vi "主函数.vi"() -> ()   [LabVIEW 2020]
doc: "UDP协议与TCP的区别在于UDP不包括发送数据包信息的错误检查，因此无法保证接收端是否已接收所发数据。\n\nUDP可用于“广播”数据至整个网络，只需指定可包括全部的IP地址(255.255.255.255)以便发送信息至整个网络。 由于路由器或其他网络硬件通常拒绝转发超过一定点的数据，在实际应用中广播范围可能存在限制。"
panel:
  in  "停止输入":bool
  out "数据状态":string
  out "当前采集数据IP地址":string
  out "输出波形":waveform(i32)[](graph)
  in  "输出文件夹名称":path
  in  "数据采集卡IP地址":string
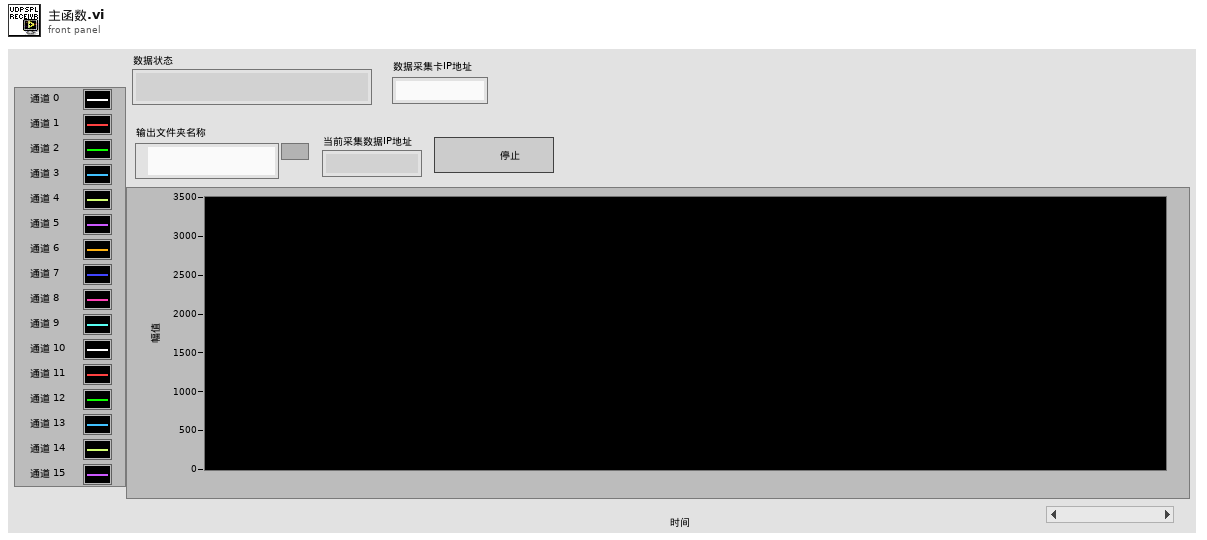
[diagram p1: front panel]
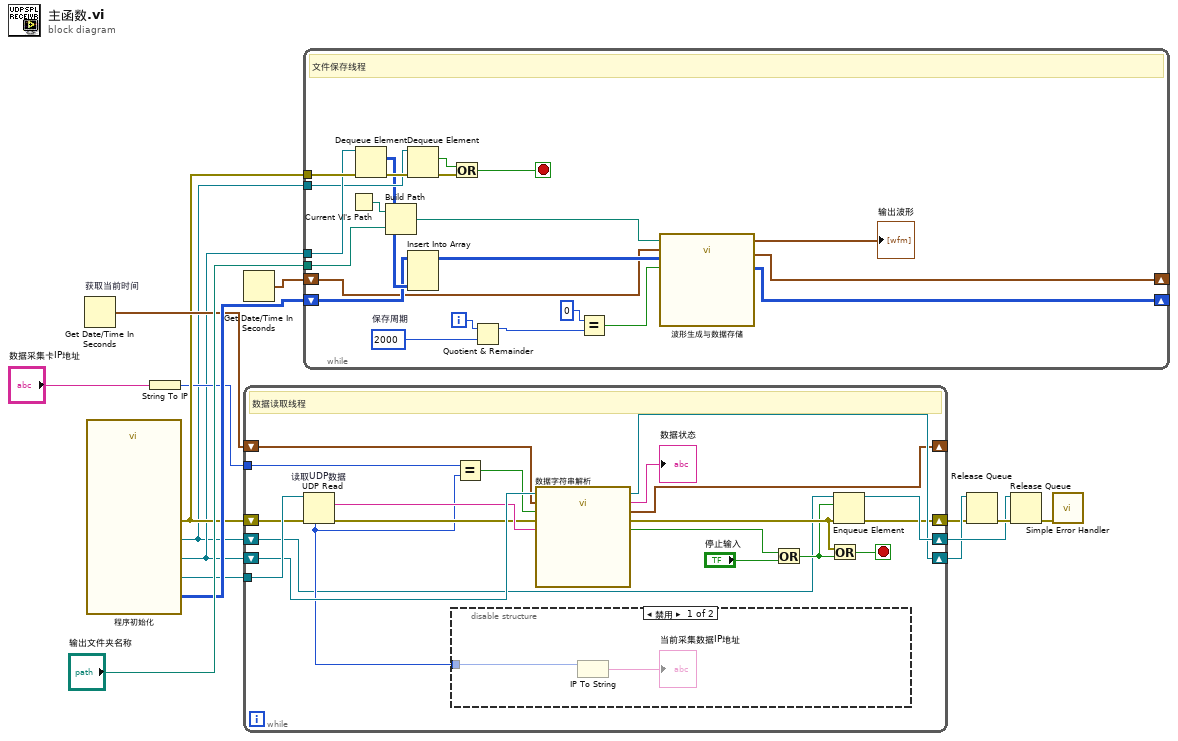
[diagram p0: block diagram]
diagram:
  n1 = Get Date/Time In Seconds "获取当前时间"() -> (seconds since 1Jan1904=w5:timestamp)
  n2 = call "程序初始化.vi"() -> ("数据传输队列"=w2:refnum<queue>, "停止位队列"=w1:refnum<queue>, "UDP网络连接输出"=w6:refnum<k16>, "error out 2"=w4:errorcluster, "初始化数组"=w13:i32[][])  [unwired: 7 in]
  n3 = String To IP(1:"数据采集卡IP地址") -> (0:w3:u32)
  n4 = Get Date/Time In Seconds() -> (seconds since 1Jan1904=w12:timestamp)
  n5 = while "While循环" {
    tunnel: w6 -> [w35]
    tunnel: w3 -> [w30]
    shift-right: [w29] -> w7
    shift-left: w4 -> [w34]
    shift-right: [w31] -> w8
    shift-left: w2 -> [w32]
    shift-right: [w33] -> w9
    shift-left: w1 -> [w16]
    shift-right: [w19] -> _
    shift-left: w5 -> [w17]
    stop <- w18 stop-if-true
    # "数据读取线程"
    n6 = UDP Read "读取UDP数据"(connection ID=w35, 8:w34) -> (data out=w28:string, error out=w24:errorcluster, 6:w20:u32)  [unwired: 1 in, 3 out]
    n7 = disable-structure shown="禁用" {
      disable-tunnel: w20 -> [w37 _]
      frame Disabled {
        n8 = IP To String(2:w37) -> (0:→"当前采集数据IP地址":string)  [unwired: 1 in]
      }
      frame Enabled {
      }
    }
    n9 = Equal?(x=w30, y=w20) -> (x = y?=w27:bool)
    n10 = call "数据字符串解析.vi"("输入数据"=w28, "错误输入（无错误）"=w24, "地址判断位"=w27, "上轮成功输入时间"=w17, "回传数据队列"=w32) -> ("错误输出"=w23:errorcluster, "输出时间"=w19:timestamp, "数据状态"=→"数据状态":string, "回传数据队列"=w31:refnum<queue>, "超时标志位"=w25:bool)  [unwired: 2 in]
    n11 = Or(x=w25, y="停止输入") -> (x .or. y?=w22:bool)
    n12 = Or(x=w23, y=w22) -> (x .or. y?=w18:bool)
    n13 = Enqueue Element(queue=w16, element=w22, error in (no error)=w23) -> (queue out=w33:refnum<queue>, error out=w29:errorcluster)  [unwired: 1 in, 1 out]
  }
  n14 = while {
    tunnel: w4 -> [w59]
    tunnel: w2 -> [w57]
    tunnel: w1 -> [w55]
    shift-right: [w44] -> _
    shift-left: w13 -> [w51]
    shift-right: [w43] -> _
    shift-left: w12 -> [w42]
    tunnel: "输出文件夹名称" -> [w39]
    i -> [w50]
    stop <- w58 stop-if-true
    w49 = 2000  # 保存周期
    # "文件保存线程"
    n15 = Current VI's Path() -> (path=w41:path)
    n16 = Dequeue Element(queue=w57, error in (no error)=w59) -> (element=w52:i32[][], error out=w56:errorcluster)  [unwired: 1 in, 2 out]
    n17 = Build Path(base path=w41, name or relative path=w39) -> (appended path=w40:path)
    n18 = Dequeue Element(queue=w55, error in (no error)=w56) -> (element=w54:bool, error out=w53:errorcluster)  [unwired: 1 in, 2 out]
    n19 = Insert Into Array(array=w51, new element=w52) -> (w45:i32[][])  [unwired: 2 in]
    n20 = Or(x=w54, y=w53) -> (x .or. y?=w58:bool)
    n21 = Quotient & Remainder(x=w50, y=w49) -> (x-y*floor(x/y)=w47:i32)  [unwired: 1 out]
    n22 = Equal?(x=0, y=w47) -> (x = y?=w46:bool)
    n23 = call "波形生成与数据存储.vi"("文件保存控制位"=w46, "数据输入"=w45, "上一时刻时间输入"=w42, "文件存储地址"=w40) -> ("缓存区输出"=w44:i32[][], "时间输出"=w43:timestamp, "输出波形"=→"输出波形":waveform(i32)[])  [unwired: 5 in]
  }
  n24 = Release Queue(queue=w8, error in (no error)=w7) -> (error out=w11:errorcluster)  [unwired: 1 in, 2 out]
  n25 = Release Queue(queue=w9, error in (no error)=w11) -> (error out=w10:errorcluster)  [unwired: 1 in, 2 out]
  n26 = call <vilib>:"Simple Error Handler.vi"("error in (no error)"=w10) -> ()  [unwired: 4 in, 5 out]
